vi "EngineStopped.vi"(10 "Engine Stopped Event Data":T1, 11 "Engine Event Interface in":refnum<class "EngineEventInterface.lvclass">) -> ()   [LabVIEW 2020, in "GLF.lvlib" / "EngineEventInterface.lvclass"]
uses:
  EngineEventInterface.lvclass
  EngineStopped-EventData--cluster.ctl
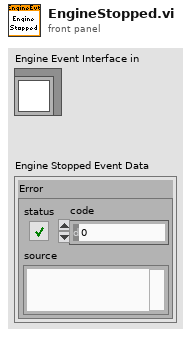
[diagram p1: front panel]
types:
  T1 = typedef "GLF.lvlib/EngineEventInterface.lvclass/EngineStopped-EventData--cluster.ctl" = cluster{"Error":errorcluster}
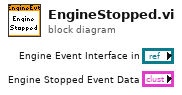
[diagram p0: block diagram]
diagram:
